vi "RTS Open TDMS.vi"(5 "Specific File Location?":bool, 7 "Chamber Number":string, 8 "error in (no error)":errorcluster, 11 "Specific File Location":path) -> (0 "Error Out":errorcluster, 1 "TDMS File Location":path, 2 "Boolean":bool, 3 "TDMS File":refnum<k34>)   [LabVIEW 2016]
panel:
  in  "Debug":bool
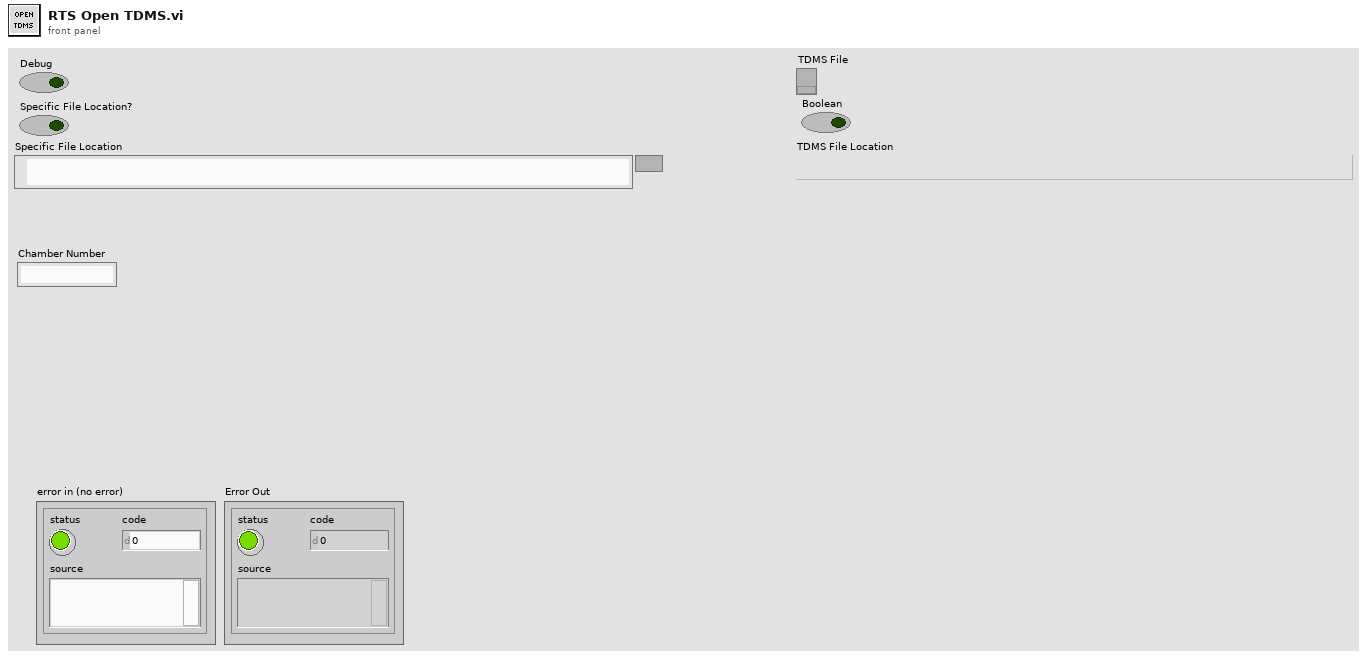
[diagram p1: front panel]
types:
  T1 = enum16{"open", "open or create", "create or replace", "create", "open (read-only)"}
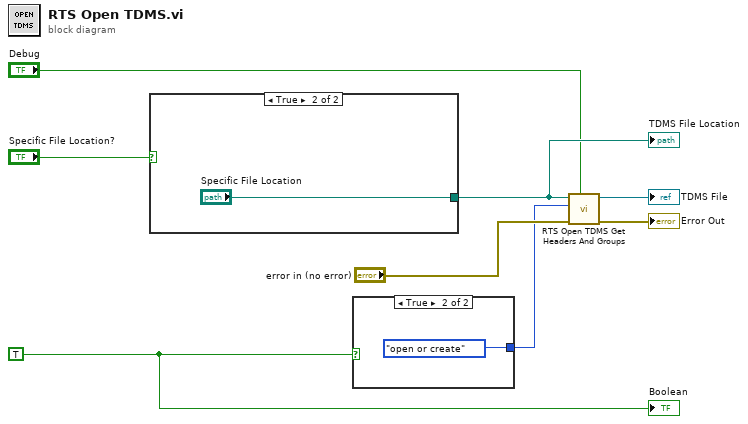
[diagram p0: block diagram]
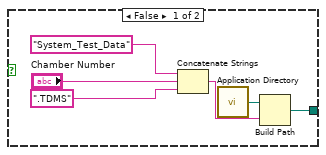
[diagram p2: hidden frame]
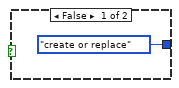
[diagram p3: hidden frame]
diagram:
  w8 = TRUE
  n1 = case shown="True" "Specific File Location?" {
    tunnel: [w9 "Specific File Location"] -> w7
    frame False {
      n2 = Concatenate Strings("System_Test_Data" ("string"), "Chamber Number", ".TDMS" ("string")) -> (w10:string)
      n3 = call <vilib>:"Application Directory.vi"() -> ("Application Directory"=w14:path)
      n4 = Build Path(base path=w14, name or relative path=w10) -> (appended path=w9:path)
    }
    frame True {
    }
  }
  "TDMS File Location" <- w7
  n5 = case shown="True" w8 {
    tunnel: [T1."create or replace" ("operation (0:open)") T1."open or create" ("operation (0:open)")] -> w5
    frame False {
    }
    frame True {
    }
  }
  n6 = call "RTS Open TDMS Get Headers And Groups.vi"("Debug"="Debug", "error in (no error)"="error in (no error)", "Operation"=w5, "file path"=w7) -> ("Error Out"=→"Error Out":errorcluster, "Refnum out"=→"TDMS File":refnum<k34>)  [unwired: 6 in]
  "Boolean" <- w8
